vi "EX1.vi"() -> ()   [LabVIEW 2018]
uses:
  <vilib>/Platform/browser.llb/Open URL in Default Browser (string).vi
panel:
  in  "Help Button":bool
  out "date/time string":string
  out "Numeric Indicator":dbl
  in  "Stop Button":bool
  in  "Initialiser":bool
  out "e":bool
  out "f":bool
  out "c":bool
  out "b":bool
  out "d":bool
  out "g":bool
  out "a":bool
  in  "Appliquer":bool
  in  "Vitesse de Comptage/Decomptage":dbl(slide) scale=1.0..10.0
  out "Mode selection":string
  in  "Comptage/Decomptage":enum32{"No Selection", "COMPTAGE", "DECOMPTAGE"}(radio)=enum."COMPTAGE"
  out "afficheur":dbl
  in  "0":bool
  in  "9":bool
  in  "8":bool
  in  "7":bool
  in  "6":bool
  in  "5":bool
  in  "4":bool
  in  "3":bool
  in  "2":bool
  in  "1":bool
  # "TP N°1"
  # "Mekni Marwen 2ème Année Génie Electrique"
  # "Exercice 1 : Comptage/decomptage/7seg"
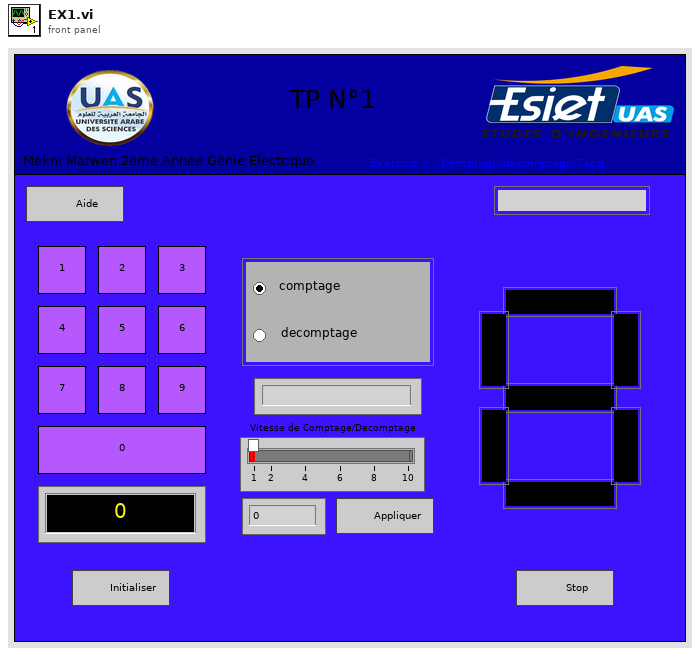
[diagram p1: front panel]
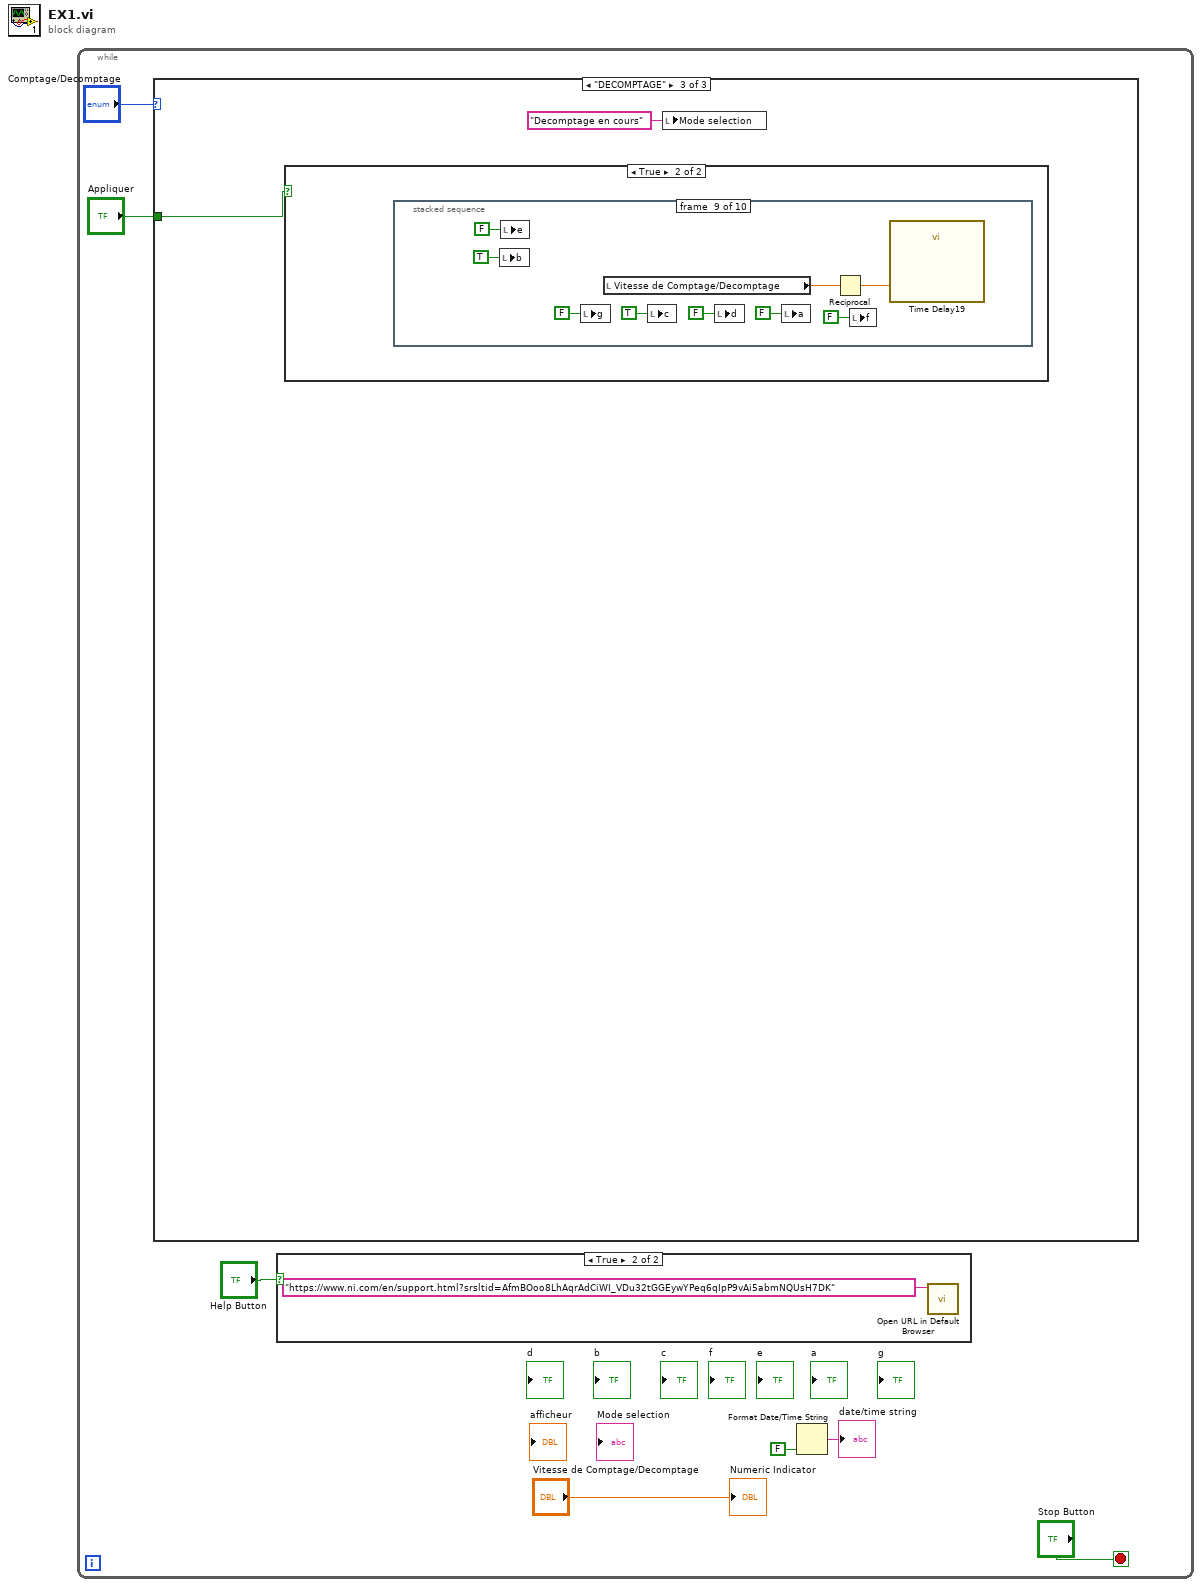
[diagram p0: block diagram]
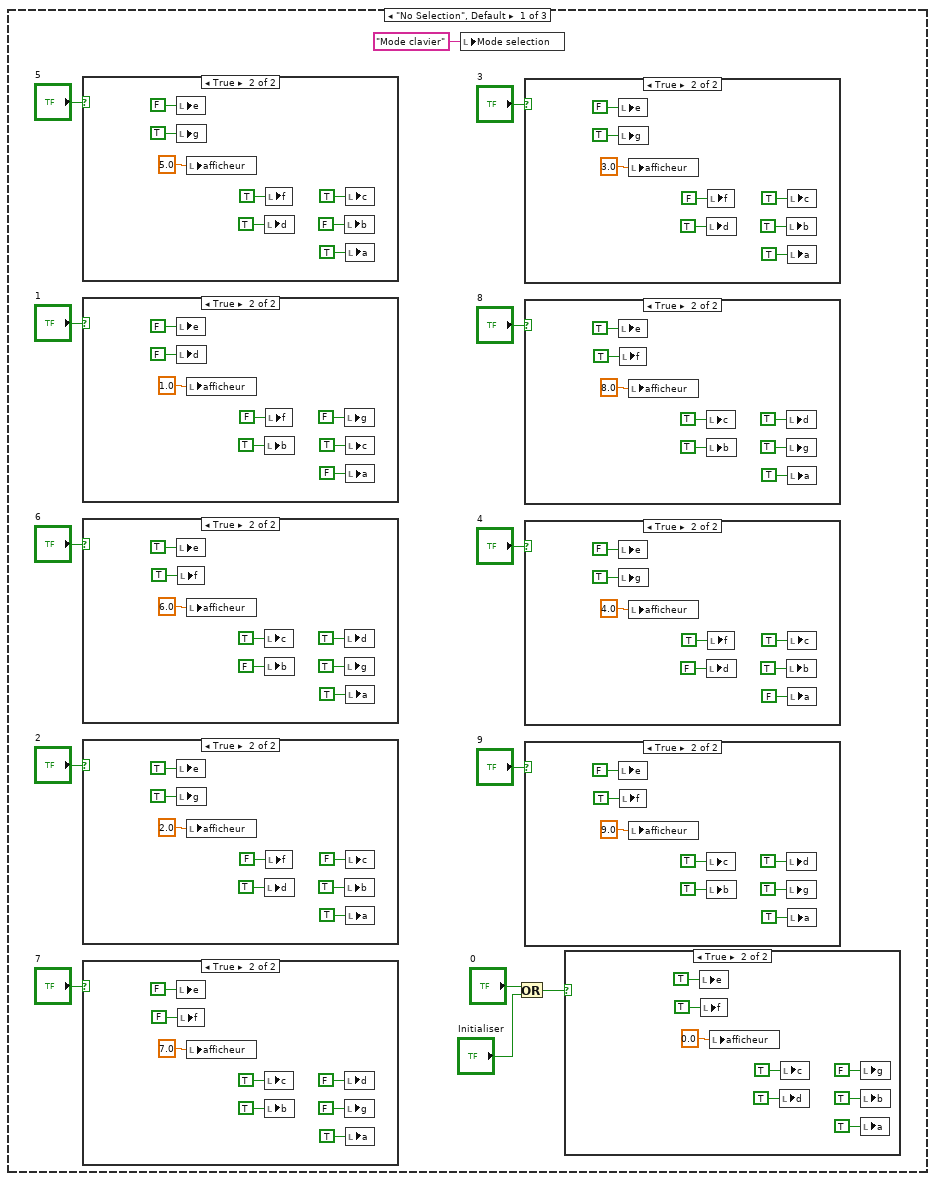
[diagram p3: hidden frame]
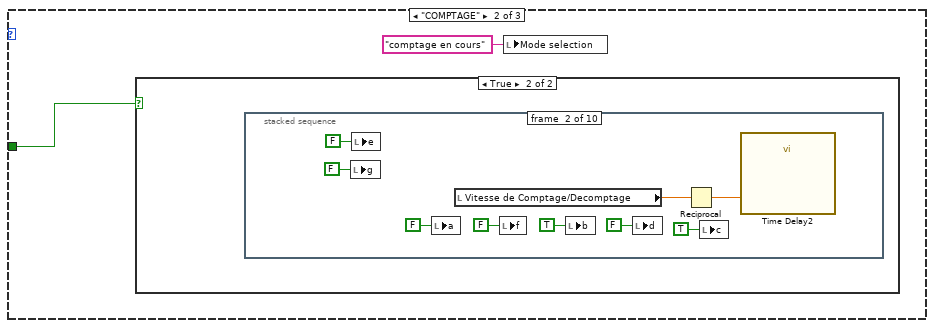
[diagram p14: hidden frame]
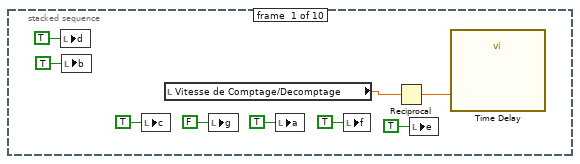
[diagram p16: hidden frame]
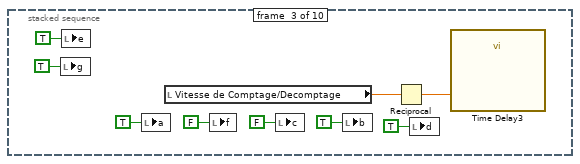
[diagram p17: hidden frame]
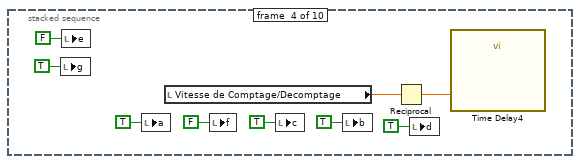
[diagram p18: hidden frame]
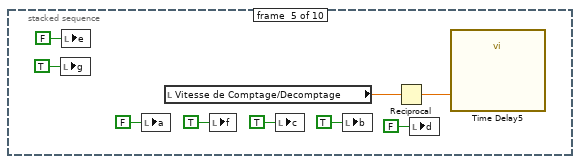
[diagram p19: hidden frame]
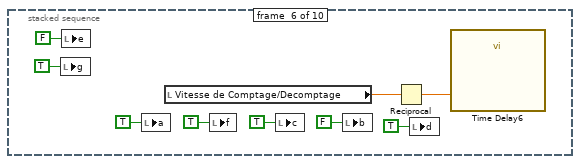
[diagram p20: hidden frame]
diagram:
  n1 = while {
    stop <- "Stop Button" stop-if-true
    n2 = case shown="\"DECOMPTAGE\"" "Comptage/Decomptage" {
      tunnel: "Appliquer" -> [_ w102 w194]
      frame "No Selection", Default {
        n3 = case shown="True" "5" {
          frame False {
          }
          frame True {
            n4 = local write "e"(FALSE ("e")) -> ()
            n5 = local write "g"(TRUE ("g")) -> ()
            n6 = local write "afficheur"(5.0 ("afficheur")) -> ()
            n7 = local write "d"(TRUE ("d")) -> ()
            n8 = local write "f"(TRUE ("f")) -> ()
            n9 = local write "b"(FALSE ("b")) -> ()
            n10 = local write "c"(TRUE ("c")) -> ()
            n11 = local write "a"(TRUE ("a")) -> ()
          }
        }
        n12 = case shown="True" "1" {
          frame False {
          }
          frame True {
            n13 = local write "e"(FALSE ("e")) -> ()
            n14 = local write "d"(FALSE ("d")) -> ()
            n15 = local write "afficheur"(1.0 ("afficheur")) -> ()
            n16 = local write "b"(TRUE ("b")) -> ()
            n17 = local write "f"(FALSE ("f")) -> ()
            n18 = local write "g"(FALSE ("g")) -> ()
            n19 = local write "c"(TRUE ("c")) -> ()
            n20 = local write "a"(FALSE ("a")) -> ()
          }
        }
        n21 = case shown="True" "6" {
          frame False {
          }
          frame True {
            n22 = local write "e"(TRUE ("e")) -> ()
            n23 = local write "f"(TRUE ("f")) -> ()
            n24 = local write "afficheur"(6.0 ("afficheur")) -> ()
            n25 = local write "c"(TRUE ("c")) -> ()
            n26 = local write "b"(FALSE ("b")) -> ()
            n27 = local write "d"(TRUE ("d")) -> ()
            n28 = local write "g"(TRUE ("g")) -> ()
            n29 = local write "a"(TRUE ("a")) -> ()
          }
        }
        n30 = case shown="True" "2" {
          frame False {
          }
          frame True {
            n31 = local write "e"(TRUE ("e")) -> ()
            n32 = local write "g"(TRUE ("g")) -> ()
            n33 = local write "afficheur"(2.0 ("afficheur")) -> ()
            n34 = local write "d"(TRUE ("d")) -> ()
            n35 = local write "f"(FALSE ("f")) -> ()
            n36 = local write "b"(TRUE ("b")) -> ()
            n37 = local write "c"(FALSE ("c")) -> ()
            n38 = local write "a"(TRUE ("a")) -> ()
          }
        }
        n39 = case shown="True" "7" {
          frame False {
          }
          frame True {
            n40 = local write "e"(FALSE ("e")) -> ()
            n41 = local write "f"(FALSE ("f")) -> ()
            n42 = local write "afficheur"(7.0 ("afficheur")) -> ()
            n43 = local write "c"(TRUE ("c")) -> ()
            n44 = local write "b"(TRUE ("b")) -> ()
            n45 = local write "d"(FALSE ("d")) -> ()
            n46 = local write "g"(FALSE ("g")) -> ()
            n47 = local write "a"(TRUE ("a")) -> ()
          }
        }
        n48 = local write "Mode selection"("Mode clavier" ("String")) -> ()
        n49 = Or(x="0", y="Initialiser") -> (x .or. y?=w11:bool)
        n50 = case shown="True" "3" {
          frame False {
          }
          frame True {
            n51 = local write "e"(FALSE ("e")) -> ()
            n52 = local write "g"(TRUE ("g")) -> ()
            n53 = local write "afficheur"(3.0 ("afficheur")) -> ()
            n54 = local write "d"(TRUE ("d")) -> ()
            n55 = local write "f"(FALSE ("f")) -> ()
            n56 = local write "b"(TRUE ("b")) -> ()
            n57 = local write "c"(TRUE ("c")) -> ()
            n58 = local write "a"(TRUE ("a")) -> ()
          }
        }
        n59 = case shown="True" "8" {
          frame False {
          }
          frame True {
            n60 = local write "e"(TRUE ("e")) -> ()
            n61 = local write "f"(TRUE ("f")) -> ()
            n62 = local write "afficheur"(8.0 ("afficheur")) -> ()
            n63 = local write "c"(TRUE ("c")) -> ()
            n64 = local write "b"(TRUE ("b")) -> ()
            n65 = local write "d"(TRUE ("d")) -> ()
            n66 = local write "g"(TRUE ("g")) -> ()
            n67 = local write "a"(TRUE ("a")) -> ()
          }
        }
        n68 = case shown="True" "4" {
          frame False {
          }
          frame True {
            n69 = local write "e"(FALSE ("e")) -> ()
            n70 = local write "g"(TRUE ("g")) -> ()
            n71 = local write "afficheur"(4.0 ("afficheur")) -> ()
            n72 = local write "d"(FALSE ("d")) -> ()
            n73 = local write "f"(TRUE ("f")) -> ()
            n74 = local write "b"(TRUE ("b")) -> ()
            n75 = local write "c"(TRUE ("c")) -> ()
            n76 = local write "a"(FALSE ("a")) -> ()
          }
        }
        n77 = case shown="True" "9" {
          frame False {
          }
          frame True {
            n78 = local write "e"(FALSE ("e")) -> ()
            n79 = local write "f"(TRUE ("f")) -> ()
            n80 = local write "afficheur"(9.0 ("afficheur")) -> ()
            n81 = local write "c"(TRUE ("c")) -> ()
            n82 = local write "b"(TRUE ("b")) -> ()
            n83 = local write "d"(TRUE ("d")) -> ()
            n84 = local write "g"(TRUE ("g")) -> ()
            n85 = local write "a"(TRUE ("a")) -> ()
          }
        }
        n86 = case shown="True" w11 {
          frame False {
          }
          frame True {
            n87 = local write "e"(TRUE ("e")) -> ()
            n88 = local write "f"(TRUE ("f")) -> ()
            n89 = local write "afficheur"(0.0 ("afficheur")) -> ()
            n90 = local write "d"(TRUE ("d")) -> ()
            n91 = local write "c"(TRUE ("c")) -> ()
            n92 = local write "g"(FALSE ("g")) -> ()
            n93 = local write "b"(TRUE ("b")) -> ()
            n94 = local write "a"(TRUE ("a")) -> ()
          }
        }
      }
      frame "COMPTAGE" {
        n95 = case shown="True" w102 {
          frame False {
          }
          frame True {
            n96 = stacked-sequence {
              frame #0 {
                n97 = local write "d"(TRUE ("d")) -> ()
                n98 = local write "b"(TRUE ("b")) -> ()
                n99 = local write "c"(TRUE ("c")) -> ()
                n100 = local read "Vitesse de Comptage/Decomptage"() -> (w105:dbl)
                n101 = local write "g"(FALSE ("g")) -> ()
                n102 = local write "a"(TRUE ("a")) -> ()
                n103 = local write "f"(TRUE ("f")) -> ()
                n104 = Reciprocal(x=w105) -> (1/x=w104:dbl)
                n105 = local write "e"(TRUE ("e")) -> ()
                n106 = call "Time Delay"("Delay Time (s)"=w104) -> ()  [unwired: 10 in, 1 out]
              }
              frame #1 {
                n107 = local write "g"(FALSE ("g")) -> ()
                n108 = local write "e"(FALSE ("e")) -> ()
                n109 = local write "a"(FALSE ("a")) -> ()
                n110 = local read "Vitesse de Comptage/Decomptage"() -> (w114:dbl)
                n111 = local write "f"(FALSE ("f")) -> ()
                n112 = local write "b"(TRUE ("b")) -> ()
                n113 = local write "d"(FALSE ("d")) -> ()
                n114 = Reciprocal(x=w114) -> (1/x=w113:dbl)
                n115 = local write "c"(TRUE ("c")) -> ()
                n116 = call "Time Delay2"("Delay Time (s)"=w113) -> ()  [unwired: 10 in, 1 out]
              }
              frame #2 {
                n117 = local write "g"(TRUE ("g")) -> ()
                n118 = local write "e"(TRUE ("e")) -> ()
                n119 = local write "a"(TRUE ("a")) -> ()
                n120 = local read "Vitesse de Comptage/Decomptage"() -> (w123:dbl)
                n121 = local write "f"(FALSE ("f")) -> ()
                n122 = local write "c"(FALSE ("c")) -> ()
                n123 = local write "b"(TRUE ("b")) -> ()
                n124 = Reciprocal(x=w123) -> (1/x=w122:dbl)
                n125 = local write "d"(TRUE ("d")) -> ()
                n126 = call "Time Delay3"("Delay Time (s)"=w122) -> ()  [unwired: 10 in, 1 out]
              }
              frame #3 {
                n127 = local write "g"(TRUE ("g")) -> ()
                n128 = local write "e"(FALSE ("e")) -> ()
                n129 = local write "a"(TRUE ("a")) -> ()
                n130 = local read "Vitesse de Comptage/Decomptage"() -> (w132:dbl)
                n131 = local write "f"(FALSE ("f")) -> ()
                n132 = local write "c"(TRUE ("c")) -> ()
                n133 = local write "b"(TRUE ("b")) -> ()
                n134 = Reciprocal(x=w132) -> (1/x=w131:dbl)
                n135 = local write "d"(TRUE ("d")) -> ()
                n136 = call "Time Delay4"("Delay Time (s)"=w131) -> ()  [unwired: 10 in, 1 out]
              }
              frame #4 {
                n137 = local write "g"(TRUE ("g")) -> ()
                n138 = local write "e"(FALSE ("e")) -> ()
                n139 = local write "a"(FALSE ("a")) -> ()
                n140 = local read "Vitesse de Comptage/Decomptage"() -> (w141:dbl)
                n141 = local write "f"(TRUE ("f")) -> ()
                n142 = local write "c"(TRUE ("c")) -> ()
                n143 = local write "b"(TRUE ("b")) -> ()
                n144 = Reciprocal(x=w141) -> (1/x=w140:dbl)
                n145 = local write "d"(FALSE ("d")) -> ()
                n146 = call "Time Delay5"("Delay Time (s)"=w140) -> ()  [unwired: 10 in, 1 out]
              }
              frame #5 {
                n147 = local write "g"(TRUE ("g")) -> ()
                n148 = local write "e"(FALSE ("e")) -> ()
                n149 = local write "a"(TRUE ("a")) -> ()
                n150 = local read "Vitesse de Comptage/Decomptage"() -> (w150:dbl)
                n151 = local write "f"(TRUE ("f")) -> ()
                n152 = local write "c"(TRUE ("c")) -> ()
                n153 = local write "b"(FALSE ("b")) -> ()
                n154 = Reciprocal(x=w150) -> (1/x=w149:dbl)
                n155 = local write "d"(TRUE ("d")) -> ()
                n156 = call "Time Delay6"("Delay Time (s)"=w149) -> ()  [unwired: 10 in, 1 out]
              }
              frame #6 {
                n157 = local write "g"(TRUE ("g")) -> ()
                n158 = local write "e"(TRUE ("e")) -> ()
                n159 = local write "a"(TRUE ("a")) -> ()
                n160 = local read "Vitesse de Comptage/Decomptage"() -> (w159:dbl)
                n161 = local write "f"(TRUE ("f")) -> ()
                n162 = local write "c"(TRUE ("c")) -> ()
                n163 = local write "b"(FALSE ("b")) -> ()
                n164 = Reciprocal(x=w159) -> (1/x=w158:dbl)
                n165 = local write "d"(TRUE ("d")) -> ()
                n166 = call "Time Delay7"("Delay Time (s)"=w158) -> ()  [unwired: 10 in, 1 out]
              }
              frame #7 {
                n167 = local write "g"(FALSE ("g")) -> ()
                n168 = local write "e"(FALSE ("e")) -> ()
                n169 = local write "a"(TRUE ("a")) -> ()
                n170 = local read "Vitesse de Comptage/Decomptage"() -> (w168:dbl)
                n171 = local write "f"(FALSE ("f")) -> ()
                n172 = local write "c"(TRUE ("c")) -> ()
                n173 = local write "b"(TRUE ("b")) -> ()
                n174 = Reciprocal(x=w168) -> (1/x=w167:dbl)
                n175 = local write "d"(FALSE ("d")) -> ()
                n176 = call "Time Delay8"("Delay Time (s)"=w167) -> ()  [unwired: 10 in, 1 out]
              }
              frame #8 {
                n177 = local write "g"(TRUE ("g")) -> ()
                n178 = local write "e"(TRUE ("e")) -> ()
                n179 = local write "a"(TRUE ("a")) -> ()
                n180 = local read "Vitesse de Comptage/Decomptage"() -> (w177:dbl)
                n181 = local write "f"(TRUE ("f")) -> ()
                n182 = local write "c"(TRUE ("c")) -> ()
                n183 = local write "b"(TRUE ("b")) -> ()
                n184 = Reciprocal(x=w177) -> (1/x=w176:dbl)
                n185 = local write "d"(TRUE ("d")) -> ()
                n186 = call "Time Delay9"("Delay Time (s)"=w176) -> ()  [unwired: 10 in, 1 out]
              }
              frame #9 {
                n187 = local write "g"(TRUE ("g")) -> ()
                n188 = local write "e"(FALSE ("e")) -> ()
                n189 = local write "a"(TRUE ("a")) -> ()
                n190 = local read "Vitesse de Comptage/Decomptage"() -> (w186:dbl)
                n191 = local write "f"(TRUE ("f")) -> ()
                n192 = local write "c"(TRUE ("c")) -> ()
                n193 = local write "b"(TRUE ("b")) -> ()
                n194 = Reciprocal(x=w186) -> (1/x=w185:dbl)
                n195 = local write "d"(TRUE ("d")) -> ()
                n196 = call "Time Delay10"("Delay Time (s)"=w185) -> ()  [unwired: 10 in, 1 out]
              }
            }
          }
        }
        n197 = local write "Mode selection"("comptage en cours" ("String")) -> ()
      }
      frame "DECOMPTAGE" {
        n198 = case shown="True" w194 {
          frame False {
          }
          frame True {
            n199 = stacked-sequence {
              frame #0 {
                n200 = local write "b"(TRUE ("b")) -> ()
                n201 = local write "e"(FALSE ("e")) -> ()
                n202 = local write "g"(TRUE ("g")) -> ()
                n203 = local read "Vitesse de Comptage/Decomptage"() -> (w197:dbl)
                n204 = local write "c"(TRUE ("c")) -> ()
                n205 = local write "d"(TRUE ("d")) -> ()
                n206 = local write "a"(TRUE ("a")) -> ()
                n207 = Reciprocal(x=w197) -> (1/x=w196:dbl)
                n208 = local write "f"(TRUE ("f")) -> ()
                n209 = call "Time Delay11"("Delay Time (s)"=w196) -> ()  [unwired: 10 in, 1 out]
              }
              frame #1 {
                n210 = local write "b"(TRUE ("b")) -> ()
                n211 = local write "e"(TRUE ("e")) -> ()
                n212 = local write "g"(TRUE ("g")) -> ()
                n213 = local read "Vitesse de Comptage/Decomptage"() -> (w206:dbl)
                n214 = local write "c"(TRUE ("c")) -> ()
                n215 = local write "d"(TRUE ("d")) -> ()
                n216 = local write "a"(TRUE ("a")) -> ()
                n217 = Reciprocal(x=w206) -> (1/x=w205:dbl)
                n218 = local write "f"(TRUE ("f")) -> ()
                n219 = call "Time Delay12"("Delay Time (s)"=w205) -> ()  [unwired: 10 in, 1 out]
              }
              frame #2 {
                n220 = local write "b"(TRUE ("b")) -> ()
                n221 = local write "e"(FALSE ("e")) -> ()
                n222 = local write "g"(FALSE ("g")) -> ()
                n223 = local read "Vitesse de Comptage/Decomptage"() -> (w215:dbl)
                n224 = local write "c"(TRUE ("c")) -> ()
                n225 = local write "d"(FALSE ("d")) -> ()
                n226 = local write "a"(TRUE ("a")) -> ()
                n227 = Reciprocal(x=w215) -> (1/x=w214:dbl)
                n228 = local write "f"(FALSE ("f")) -> ()
                n229 = call "Time Delay13"("Delay Time (s)"=w214) -> ()  [unwired: 10 in, 1 out]
              }
              frame #3 {
                n230 = local write "b"(FALSE ("b")) -> ()
                n231 = local write "e"(TRUE ("e")) -> ()
                n232 = local write "g"(TRUE ("g")) -> ()
                n233 = local read "Vitesse de Comptage/Decomptage"() -> (w224:dbl)
                n234 = local write "c"(TRUE ("c")) -> ()
                n235 = local write "d"(TRUE ("d")) -> ()
                n236 = local write "a"(TRUE ("a")) -> ()
                n237 = Reciprocal(x=w224) -> (1/x=w223:dbl)
                n238 = local write "f"(TRUE ("f")) -> ()
                n239 = call "Time Delay14"("Delay Time (s)"=w223) -> ()  [unwired: 10 in, 1 out]
              }
              frame #4 {
                n240 = local write "b"(FALSE ("b")) -> ()
                n241 = local write "e"(FALSE ("e")) -> ()
                n242 = local write "g"(TRUE ("g")) -> ()
                n243 = local read "Vitesse de Comptage/Decomptage"() -> (w233:dbl)
                n244 = local write "c"(TRUE ("c")) -> ()
                n245 = local write "d"(TRUE ("d")) -> ()
                n246 = local write "a"(TRUE ("a")) -> ()
                n247 = Reciprocal(x=w233) -> (1/x=w232:dbl)
                n248 = local write "f"(TRUE ("f")) -> ()
                n249 = call "Time Delay15"("Delay Time (s)"=w232) -> ()  [unwired: 10 in, 1 out]
              }
              frame #5 {
                n250 = local write "b"(TRUE ("b")) -> ()
                n251 = local write "e"(FALSE ("e")) -> ()
                n252 = local write "g"(TRUE ("g")) -> ()
                n253 = local read "Vitesse de Comptage/Decomptage"() -> (w242:dbl)
                n254 = local write "c"(TRUE ("c")) -> ()
                n255 = local write "d"(FALSE ("d")) -> ()
                n256 = local write "a"(FALSE ("a")) -> ()
                n257 = Reciprocal(x=w242) -> (1/x=w241:dbl)
                n258 = local write "f"(TRUE ("f")) -> ()
                n259 = call "Time Delay17"("Delay Time (s)"=w241) -> ()  [unwired: 10 in, 1 out]
              }
              frame #6 {
                n260 = local write "b"(TRUE ("b")) -> ()
                n261 = local write "e"(FALSE ("e")) -> ()
                n262 = local write "g"(TRUE ("g")) -> ()
                n263 = local read "Vitesse de Comptage/Decomptage"() -> (w251:dbl)
                n264 = local write "c"(TRUE ("c")) -> ()
                n265 = local write "d"(TRUE ("d")) -> ()
                n266 = local write "a"(TRUE ("a")) -> ()
                n267 = Reciprocal(x=w251) -> (1/x=w250:dbl)
                n268 = local write "f"(FALSE ("f")) -> ()
                n269 = call "Time Delay16"("Delay Time (s)"=w250) -> ()  [unwired: 10 in, 1 out]
              }
              frame #7 {
                n270 = local write "b"(TRUE ("b")) -> ()
                n271 = local write "e"(TRUE ("e")) -> ()
                n272 = local write "g"(TRUE ("g")) -> ()
                n273 = local read "Vitesse de Comptage/Decomptage"() -> (w260:dbl)
                n274 = local write "c"(FALSE ("c")) -> ()
                n275 = local write "d"(TRUE ("d")) -> ()
                n276 = local write "a"(TRUE ("a")) -> ()
                n277 = Reciprocal(x=w260) -> (1/x=w259:dbl)
                n278 = local write "f"(FALSE ("f")) -> ()
                n279 = call "Time Delay18"("Delay Time (s)"=w259) -> ()  [unwired: 10 in, 1 out]
              }
              frame #8 {
                n280 = local write "b"(TRUE ("b")) -> ()
                n281 = local write "e"(FALSE ("e")) -> ()
                n282 = local write "g"(FALSE ("g")) -> ()
                n283 = local read "Vitesse de Comptage/Decomptage"() -> (w269:dbl)
                n284 = local write "c"(TRUE ("c")) -> ()
                n285 = local write "d"(FALSE ("d")) -> ()
                n286 = local write "a"(FALSE ("a")) -> ()
                n287 = Reciprocal(x=w269) -> (1/x=w268:dbl)
                n288 = local write "f"(FALSE ("f")) -> ()
                n289 = call "Time Delay19"("Delay Time (s)"=w268) -> ()  [unwired: 10 in, 1 out]
              }
              frame #9 {
                n290 = local write "b"(TRUE ("b")) -> ()
                n291 = local write "e"(TRUE ("e")) -> ()
                n292 = local write "g"(FALSE ("g")) -> ()
                n293 = local read "Vitesse de Comptage/Decomptage"() -> (w278:dbl)
                n294 = local write "c"(TRUE ("c")) -> ()
                n295 = local write "d"(TRUE ("d")) -> ()
                n296 = local write "a"(TRUE ("a")) -> ()
                n297 = Reciprocal(x=w278) -> (1/x=w277:dbl)
                n298 = local write "f"(TRUE ("f")) -> ()
                n299 = call "Time Delay20"("Delay Time (s)"=w277) -> ()  [unwired: 10 in, 1 out]
              }
            }
          }
        }
        n300 = local write "Mode selection"("Decomptage en cours" ("String")) -> ()
      }
    }
    n301 = case shown="True" "Help Button" {
      frame False {
      }
      frame True {
        n302 = call-poly <vilib>:"Open URL in Default Browser.vi"("URL"="https://www.ni.com/en/support.html?srsltid=AfmBOoo8LhAqrAdCiWI_VDu32tGGEywYPeq6qIpP9vAi5abmNQUsH7DK") -> ()  [unwired: 5 in, 2 out]
      }
    }
    n303 = Format Date/Time String(UTC format=FALSE) -> (date/time string=→"date/time string":string)  [unwired: 2 in]
    "Numeric Indicator" <- "Vitesse de Comptage/Decomptage"
  }
